vi "HTML Report.vi"(0 "report file path":path, 1 "Column Headers":string[](array[string]), 2 "Header":string="Example Report with Images", 7 "Table Data":string[][](array[string]), 11 "error in (no error)":errorcluster) -> (15 "error out":errorcluster)   [LabVIEW 2017]
doc: "This is an example of some of the things that you can do with HTML reports."
uses:
  <vilib>/Utility/NIReport.llb/Append Text Table to Report (wrap).vi
  <vilib>/printing/OpenHTMLReport.llb/Open HTML Report in Browser (Refnum).vi
  <vilib>/Utility/NIReport.llb/NI_report.lvclass
  <vilib>/Utility/NIReport.llb/NI_ReportGenerationCore.lvlib
panel:
  in  "Summary":string[](array[string])
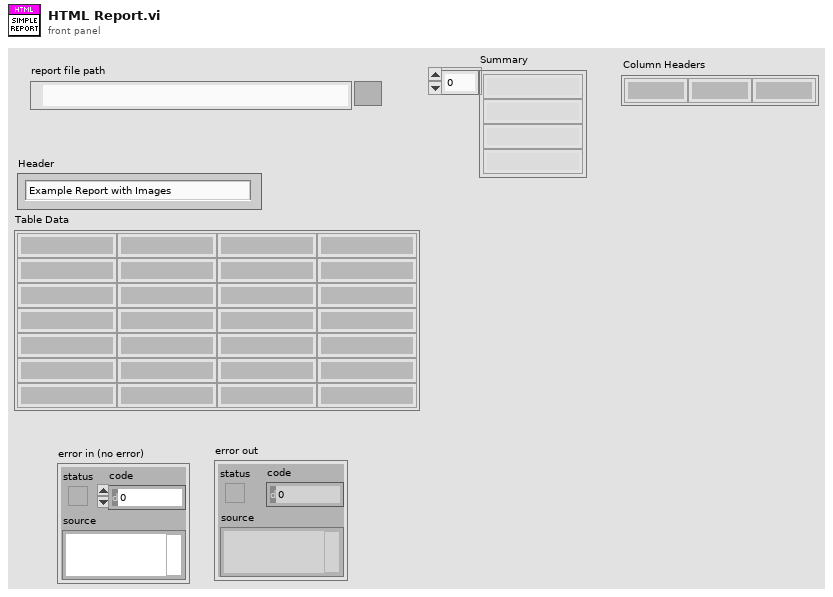
[diagram p1: front panel]
types:
  T1 = enum16{"Standard Report", "HTML", "Word", "Excel"}
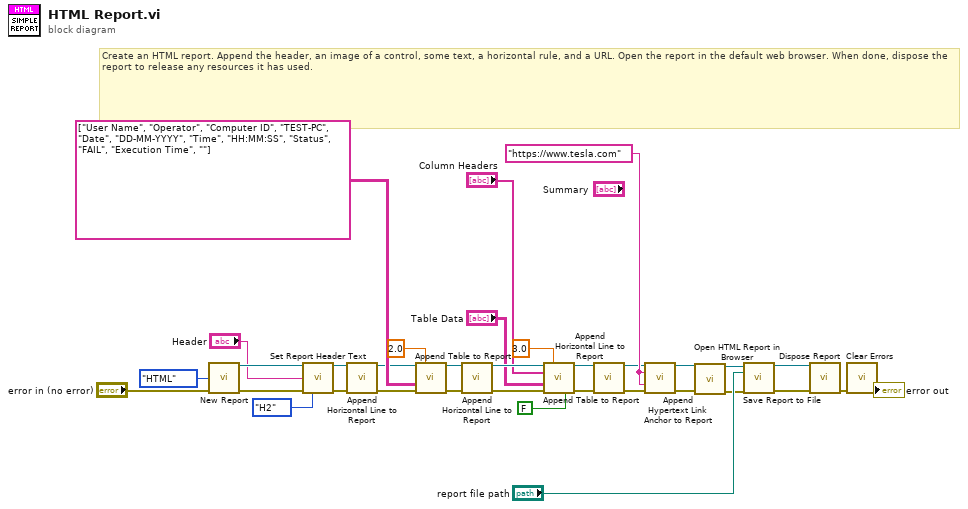
[diagram p0: block diagram]
diagram:
  w34 = "https://www.tesla.com" ("URL of link - href")
  # "Create an HTML report. Append the header, an image of a control, some text, a horizontal rule, and a URL. Open the report in the default web browser. When done, dispose the report to release any resources it has used."
  n1 = call <vilib>:"New Report.vi"("report type"=T1."HTML", "error in (no error)"="error in (no error)") -> ("report out"=w32:refnum<class "NI_report.lvclass">, "error out"=w33:errorcluster)  [unwired: 12 in]
  n2 = call-dynamic "Set Report Header Text.vi"("report in"=w32, "center header text"="Header", "error in (no error)"=w33, "HTML header size"=enum16{"H1", "H2", "H3", "H4", "H5", "H6", "H7"}."H2") -> ("report out"=w26:refnum<class "NI_report.lvclass">, "error out"=w25:errorcluster)  [unwired: 10 in]
  n3 = call-dynamic "Append Horizontal Line to Report.vi"("report in"=w26, "error in (no error)"=w25) -> ("report out"=w19:refnum<class "NI_report.lvclass">, "error out"=w24:errorcluster)  [unwired: 12 in]
  n4 = call-poly <vilib>:"Append Table to Report.vi"("report in"=w19, "column width (1)"=2.0, "text data"=string[][] [["User Name", "Operator"], ["Computer ID", "TEST-PC"], ["Date", "DD-MM-YYYY"], ["Time", "HH:MM:SS"], ["Status", "FAIL"], ["Execution Time", ""]], "error in (no error)"=w24) -> ("report out"=w20:refnum<class "NI_report.lvclass">, "error out"=w22:errorcluster)  [unwired: 8 in, 2 out]
  n5 = call-dynamic "Append Horizontal Line to Report.vi"("report in"=w20, "error in (no error)"=w22) -> ("report out"=w21:refnum<class "NI_report.lvclass">, "error out"=w17:errorcluster)  [unwired: 12 in]
  n6 = call-poly <vilib>:"Append Table to Report.vi"("report in"=w21, "column width (1)"=3.0, "column headers"="Column Headers", "text data"="Table Data", "error in (no error)"=w17, "show grid lines (YES)"=FALSE) -> ("report out"=w15:refnum<class "NI_report.lvclass">, "error out"=w16:errorcluster)  [unwired: 6 in, 2 out]
  n7 = call-dynamic "Append Horizontal Line to Report.vi"("report in"=w15, "error in (no error)"=w16) -> ("report out"=w28:refnum<class "NI_report.lvclass">, "error out"=w27:errorcluster)  [unwired: 12 in]
  n8 = call-dynamic "Append Hypertext Link Anchor to Report.vi"("report in"=w28, "URL of link - href"=w34, "link text"=w34, "error in (no error)"=w27) -> ("report out"=w4:refnum<class "NI_report.lvclass">, "error out"=w3:errorcluster)  [unwired: 8 in, 2 out]
  n9 = call-poly <vilib>:"Open HTML Report in Browser.vi"("report in"=w4, "error in (no error)"=w3) -> ("report out"=w2:refnum<class "NI_report.lvclass">, "error out"=w1:errorcluster)  [unwired: 11 in, 1 out]
  n10 = call-dynamic "Save Report to File.vi"("report in"=w2, "report file path"="report file path", "error in (no error)"=w1) -> ("report out"=w8:refnum<class "NI_report.lvclass">, "error out"=w6:errorcluster)  [unwired: 11 in]
  n11 = call-dynamic "Dispose Report.vi"("report in"=w8, "error in (no error)"=w6) -> ("error out"=w9:errorcluster)  [unwired: 13 in]
  n12 = call <vilib>:"Clear Errors.vi"("error in (no error)"=w9) -> ("error out"=→"error out":errorcluster)  [unwired: 5 in, 1 out]
